vi "getReadFile.vi"(1 "Folder Path":path) -> (0 "error out":errorcluster)   [LabVIEW 2017]
uses:
  Globals/measurementGlobal.vi
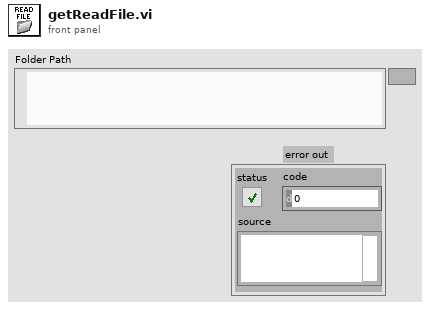
[diagram p1: front panel]
types:
  T1 = typedef "chan&Span.ctl" = cluster{"Chan No.":i32, "Low Volt Limit (-10V)":dbl, "High Volt Limit (10V)":dbl, "input terminal configuration":i32}
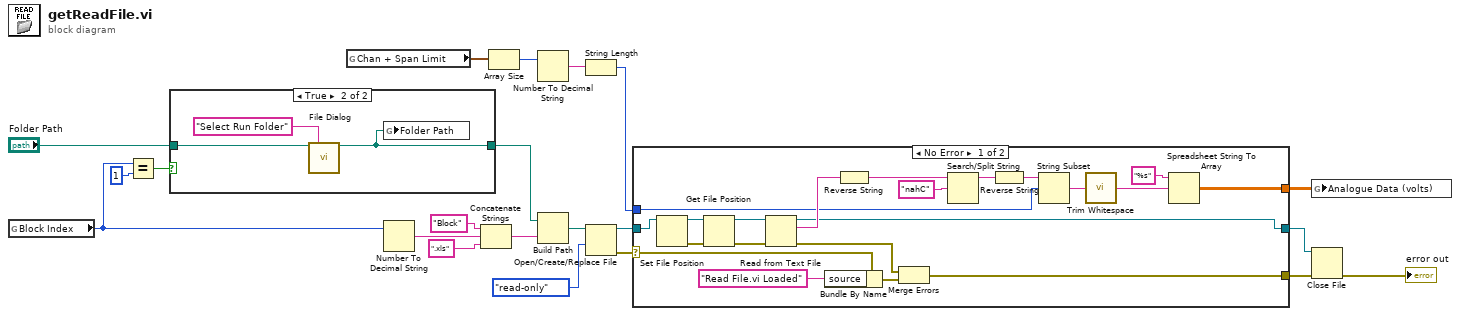
[diagram p0: block diagram]
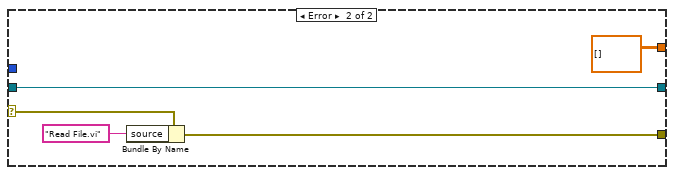
[diagram p3: hidden frame]
diagram:
  n1 = global read "measurementGlobal.vi" "Block Index"() -> (w8:i32)
  n2 = Equal?(x=w8, y=1) -> (x = y?=w6:bool)
  n3 = case shown="True" w6 {
    tunnel: "Folder Path" -> [w22 w25]
    tunnel: [w22 w23] -> w14
    frame False {
    }
    frame True {
      n4 = call "File Dialog"("start path"=w25, "prompt"="Select Run Folder") -> ("selected path"=w23:path)  [unwired: 10 in, 3 out]
      n5 = global write "measurementGlobal.vi" "Folder Path"(w23) -> ()
    }
  }
  n6 = global read "measurementGlobal.vi" "Chan + Span Limit"() -> (w4:T1[])
  n7 = Number To Decimal String(number=w8) -> (decimal integer string=w11:string)  [unwired: 1 in]
  n8 = Concatenate Strings("Block" ("name or relative path"), w11, ".xls" ("name or relative path")) -> (w9:string)
  n9 = Array Size(array=w4) -> (size(s)=w2:i32)
  n10 = Number To Decimal String(number=w2) -> (decimal integer string=w3:string)  [unwired: 1 in]
  n11 = Build Path(base path=w14, name or relative path=w9) -> (appended path=w13:path)
  n12 = String Length(string=w3) -> (length=w1:i32)
  n13 = Open/Create/Replace File(file path (use dialog)=w13, access (0:read/write)=enum16{"read/write", "read-only", "write-only"}."read-only") -> (refnum out=w20:refnum<file>, error out=w16:errorcluster)  [unwired: 4 in, 1 out]
  n14 = case shown="No Error" w16 {
    selector: w16 -> [w33 w48]
    tunnel: w20 -> [w46 w51]
    tunnel: [w27 w51] -> w19
    tunnel: [w30 w47] -> w18
    tunnel: [w29 dbl[][] []] -> w15
    tunnel: w1 -> [w26 _]
    frame No Error {
      n15 = Set File Position(refnum=w46) -> (refnum out=w45:refnum<file>, error out=w44:errorcluster)  [unwired: 3 in]
      n16 = Get File Position(4:w44, 7:w45) -> (0:w43:errorcluster, 3:w42:refnum<file>)  [unwired: 1 out]
      n17 = Read from Text File(file (use dialog)=w42, error in=w43) -> (refnum out=w27:refnum<file>, text=w41:string, error out=w28:errorcluster)  [unwired: 2 in, 1 out]
      n18 = Bundle By Name(cluster=w33, "source"="Read File.vi Loaded") -> (w31:errorcluster)
      n19 = Reverse String(1:w41) -> (0:w40:string)
      n20 = Merge Errors(w28, w31) -> (w30:errorcluster)
      n21 = Search/Split String(string=w40, search string/char (-)="nahC") -> (substring before match=w38:string)  [unwired: 1 in, 2 out]
      n22 = Reverse String(1:w38) -> (0:w37:string)
      n23 = String Subset(string=w37, offset (0)=w26) -> (substring=w35:string)  [unwired: 1 in]
      n24 = call <vilib>:"Trim Whitespace.vi"("string"=w35) -> ("trimmed string"=w34:string)  [unwired: 1 in]
      n25 = Spreadsheet String To Array(format string="%s", spreadsheet string=w34) -> (array=w29:dbl[][])  [unwired: 2 in]
    }
    frame Error {
      n26 = Bundle By Name(cluster=w48, "source"="Read File.vi") -> (w47:errorcluster)
    }
  }
  n27 = global write "measurementGlobal.vi" "Analogue Data (volts)"(w15) -> ()
  n28 = Close File(refnum=w19, error in=w18) -> (error out=→"error out":errorcluster)  [unwired: 1 out]
